vi "CS-4 Error Message.vi"(8 "error in (no error)":errorcluster, 10 "Type of Dialog (1: OK Msg)":i32(ring)=1 items=["No Dialog", "OK Message", "Continue or Stop Message"], 11 "VISA session":refnum<visa-resource-name>) -> (0 "error out":errorcluster, 1 "Error Message (empty)":string, 2 "Error Code (0)":i32, 3 "dup VISA session":refnum<visa-resource-name>, 7 "Status":bool)   [LabVIEW 2016]
doc: "CS-4 Error Msg.vi interprets CS-4 error codes. The following error codes are defined:\n\n -1301: \"CS-4 Execution Error\" occurs when a command recognized by the CS-4 command parser can not be executed. This may be the result of a controlling command being sent while in menu mode or a bad command parameter. \n -1302: \"CS-4 Command Error\" occurs if an invalid command or a command with an invalid parameter is received by the CS-4.\n -1303: \"Undefined Error\" is not presently used.\n -1304: \"CS-4 Query Error\" is generated under the conditions specified in IEEE Std 488.2-1992.\n -1305: \"CS-4 in Local or Menu\" will occur when a remote command is sent to the CS-4 while the operator has Local selected or is using the menu system."
panel:
  in  "User-Defined Descriptions":string[](array[string])=["CS-4 Execution Error", "CS-4 Command Error", "Undefined Error", "CS-4 Query Error", "CS-4 in Menu or Local mode"]
  in  "User-Defined Codes":i32[](array[numeric])=[-1301, -1302, -1303, -1304, -1305] format="%.0x"
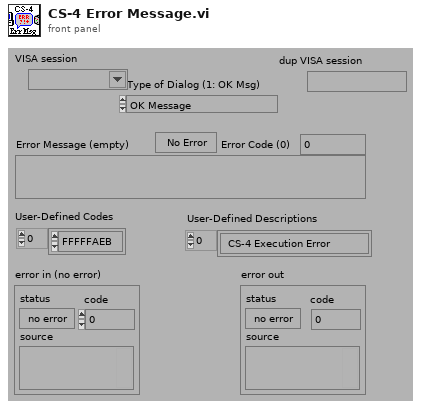
[diagram p1: front panel]
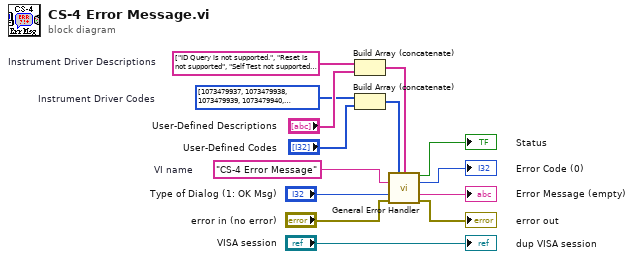
[diagram p0: block diagram]
diagram:
  w3 = i32[] [1073479937, 1073479938, 1073479939, 1073479940, 1073479941]  # Instrument Driver Codes
  w6 = string[] ["ID Query is not supported.", "Reset is not supported", "Self Test not supported.", "Error Query not supported.", "Revision Query not supported."]  # Instrument Driver Descriptions
  w11 = "CS-4 Error Message"  # VI name
  n1 = Build Array (concatenate)(w6, "User-Defined Descriptions") -> (w2:string[])
  n2 = Build Array (concatenate)(w3, "User-Defined Codes") -> (w1:i32[])
  n3 = call <vilib>:"General Error Handler.vi"("[user-defined codes]"=w1, "[user-defined descriptions]"=w2, "[error source] (\" \")"=w11, "type of dialog (OK msg:1)"="Type of Dialog (1: OK Msg)", "error in (no error)"="error in (no error)") -> ("error?"=→"Status":bool, "code out"=→"Error Code (0)":i32, "message"=→"Error Message (empty)":string, "error out"=→"error out":errorcluster)  [unwired: 6 in, 1 out]
  "dup VISA session" <- "VISA session"
